vi "Get_Coh_Control_Status.vi"(8 "error in (no error)":errorcluster, 11 ".NET Reference in":refnum<k24>) -> (0 "error out":errorcluster, 2 "status":enum16{"Coh_OFF", "Coh_ON", ""}(ring), 3 "Reference out":refnum<k24>)   [LabVIEW 2017]
uses:
  C:/Users/Ssantec_Test/Documents/Instrument_DLL_Sample_Labview_20220902_Ver1.2.2/DLL/x86/InstrumentDLL.dll
  DLL/x86/InstrumentDLL.dll
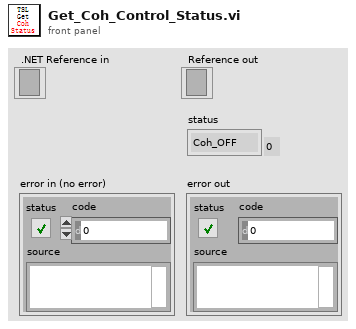
[diagram p1: front panel]
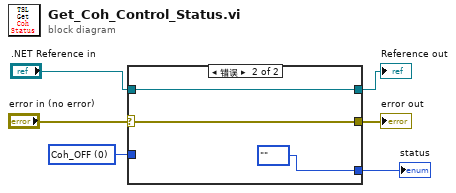
[diagram p0: block diagram]
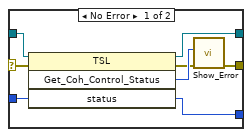
[diagram p2: hidden frame]
diagram:
  w3 = 0 items=["Coh_OFF", "Coh_ON"] ("status")
  n1 = case shown="错误" "error in (no error)" {
    selector: "error in (no error)" -> [w8 w16]
    tunnel: ".NET Reference in" -> [w14 w17]
    tunnel: [w13 w17] -> w5
    tunnel: [w9 w16] -> w4
    tunnel: w3 -> [w12 _]
    tunnel: [w7 enum16{"Coh_OFF", "Coh_ON", ""}."" ("status")] -> w1
    frame No Error {
      n2 = invoke on="调用节点" class="TSL" method="Get_Coh_Control_Status"(reference=w14, error in=w8, "status"=w12) -> (reference out=w13:refnum<k24>, error out=w10:errorcluster, "Get_Coh_Control_Status"=w11:i32, "status"=w7:i32)  [unwired: 1 in]
      n3 = call "Show_Error.vi"("error in (no error)"=w10, "Error"=w11) -> ("error out"=w9:errorcluster)  [unwired: 9 in]
    }
    frame Error {
    }
  }
  "Reference out" <- w5
  "error out" <- w4
  "status" <- w1
